vi "clear_core_data.vi"(8 "error in (no error)":errorcluster) -> (0 "error out":errorcluster)   [LabVIEW 2018, in "core.lvlib" / "core_data.lvlib"]
uses:
  core_data.lvlib
panel:
  # "Development\ncontrols/indicators useful for development and testing, but which are not outputs of the VI"
  # "Input\nInputs to the VI"
  # "Output\nOutputs of the VI"
  # "Description\n\nBlank VI with error handling case. \n\nSummarize the use of this VI in this space."
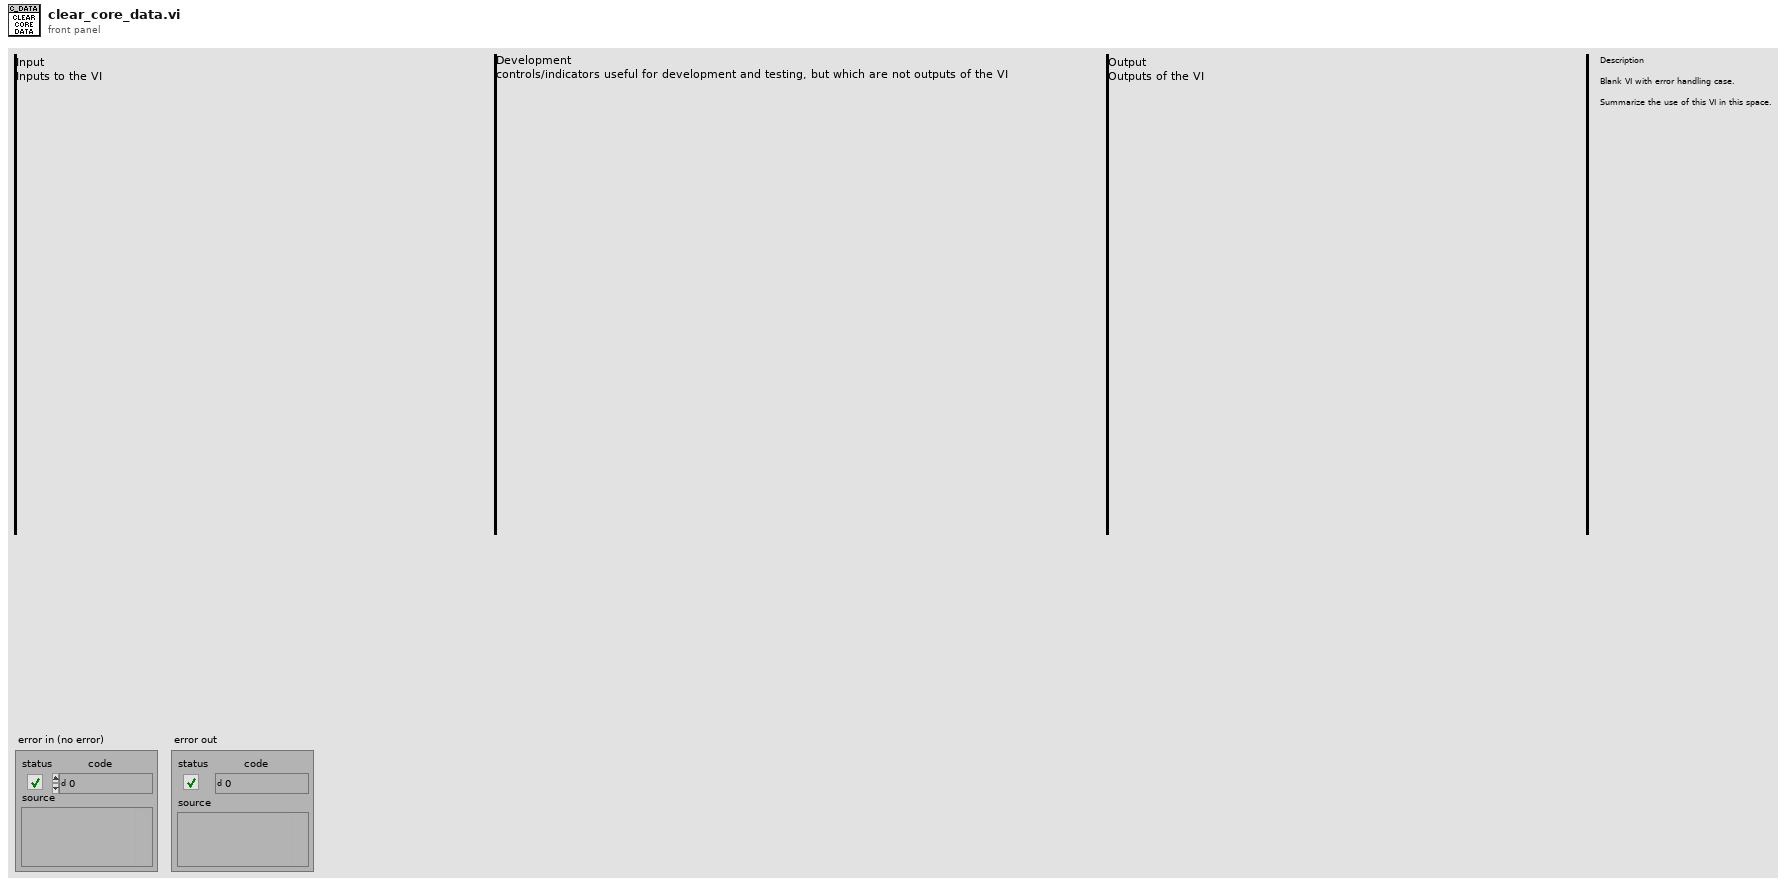
[diagram p1: front panel]
types:
  T1 = typedef "core.lvlib/core_data.lvlib/core_data.ctl" = cluster{"tour_in_progress":T2, "total no. of moves forward":u64, "total no. of moves backward":u64, "chessboard":T4[][], "square_to_move_forward_to":T3}
  T2 = typedef "core.lvlib/core_data.lvlib/tour_in_progress.ctl" = cluster{"start_time":timestamp, "tour":T3[], "no. of moves forward":u64, "no. of moves backward":u64}
  T3 = typedef "core.lvlib/core_data.lvlib/chessboard_index.ctl" = cluster{"row":u8, "column":u8}
  T4 = typedef "core.lvlib/core_data.lvlib/chess_square.ctl" = cluster{"Explored?":bool, "neighbouring_squares":T5[]}
  T5 = typedef "core.lvlib/core_data.lvlib/neighbour_square.ctl" = cluster{"row":u8, "column":u8, "exhausted?":bool}
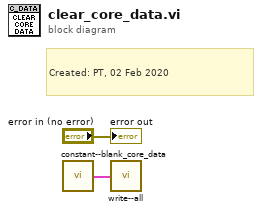
[diagram p0: block diagram]
diagram:
  # "Created: PT, 02 Feb 2020"
  n1 = call "constant--blank_core_data.vi"() -> ("blank core_data"=w2:T1)
  n2 = call "write--all.vi"("core_data"=w2) -> ()
  "error out" <- "error in (no error)"
